vi "RemoveTripleQuotes.vi"(11 "Python Code in":string) -> (3 "Python Code out":string)   [LabVIEW 2022 SP3]
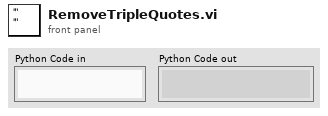
[diagram p1: front panel]
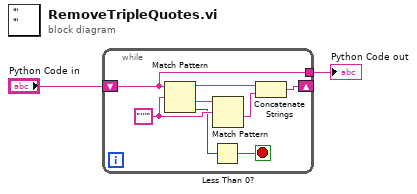
[diagram p0: block diagram]
diagram:
  n1 = while {
    shift-right: [w7] -> _
    shift-left: "Python Code in" -> [w3]
    tunnel: [w3] -> w2
    stop <- w4 stop-if-true
    w6 = "'''" ("regular expression")
    n2 = Match Pattern(string=w3, regular expression=w6) -> (before substring=w8:string, after substring=w10:string, offset past match=w5:i32)  [unwired: 1 in, 1 out]
    n3 = Less Than 0?(x=w5) -> (x < 0?=w4:bool)
    n4 = Match Pattern(string=w10, regular expression=w6) -> (after substring=w9:string)  [unwired: 1 in, 3 out]
    n5 = Concatenate Strings(w8, w9) -> (w7:string)
  }
  "Python Code out" <- w2
